vi "ZHLEDCRC-16山推.vi"(11 "String":string) -> (1 "CRC-16":u16 format="%x", 2 "CRC-16":string, 3 "String & CRC-16":string)   [LabVIEW 2016]
panel:
  out "FFFF(U16)":u16 format="%x"
  # "VI Name: MB CRC-16.vi\nPurpose: Computes the CRC of a string.\nReentrant VI, because its caller is also reentrant."
  # "CRC低字节在前，高字节在后"
  # "00010120000100020003000400050006000700080009000100020003000000010000000200010002 CD FB"
  # "$00989680010104030300000000000000000000000000000000000000000000000000000001000000000000000000950AA70000000001010C010161F0"
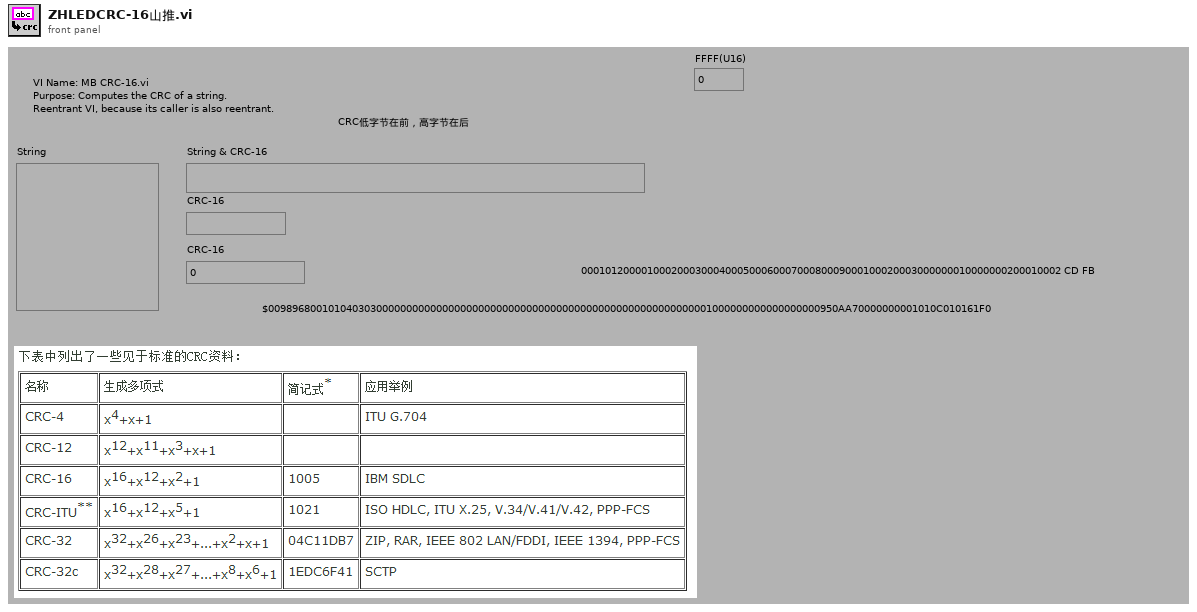
[diagram p1: front panel]
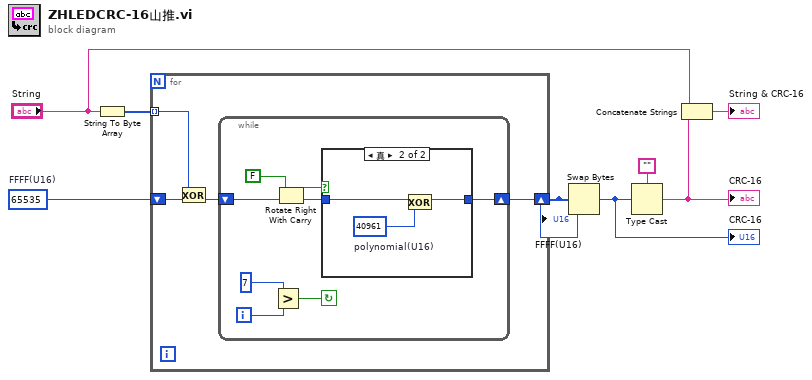
[diagram p0: block diagram]
diagram:
  w4 = u16 65535  # FFFF(U16)
  n1 = String To Byte Array(string="String") -> (unsigned byte array=w2:u8[])
  n2 = for {
    tunnel: w2 -> [w12] mode=indexing
    shift-right: [w9] -> w3
    shift-left: w4 -> [w11]
    n3 = Exclusive Or(1:w11, 2:w12) -> (0:w10:u16)
    n4 = while {
      shift-right: [w16] -> w9
      shift-left: w10 -> [w14]
      i -> [w15]
      stop <- w13 continue-if-true
      n5 = Greater?(x=7, y=w15) -> (0:w13:bool)
      n6 = Rotate Right With Carry(2:w14, 3:FALSE) -> (0:w17:u16, 1:w18:bool)
      n7 = case shown="真" w18 {
        tunnel: w17 -> [w21 w24]
        tunnel: [w21 w22] -> w16
        frame False {
        }
        frame True {
          w23 = u16 40961  # polynomial(U16)
          n8 = Exclusive Or(1:w23, 2:w24) -> (0:w22:u16)
        }
      }
    }
  }
  "FFFF(U16)" <- w3
  n9 = Swap Bytes(anything=w3) -> (byte swapped=w8:u16)
  "CRC-16" <- w8
  n10 = Type Cast(type="", x=w8) -> (*(type *) &x=w6:string)
  "CRC-16" <- w6
  n11 = Concatenate Strings("String", w6) -> (→"String & CRC-16":string)
